vi "Insert Panel to Subpanel.vi"(7 "SubPanel in":refnum<vi>, 8 "error in":errorcluster, 11 "VI Ref":refnum<vi>) -> (0 "error out":errorcluster)   [LabVIEW 2021]
doc: "This vi helps to insert graph or chart vi ref into a subpanel."
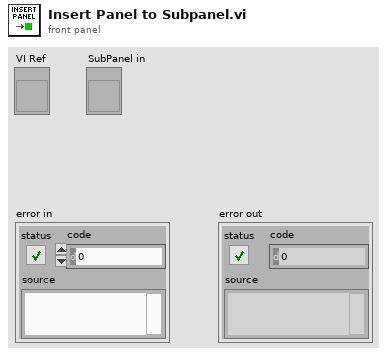
[diagram p1: front panel]
types:
  T1 = enum32{"Invalid", "Standard", "Closed", "Hidden", "Minimized", "Maximized"}
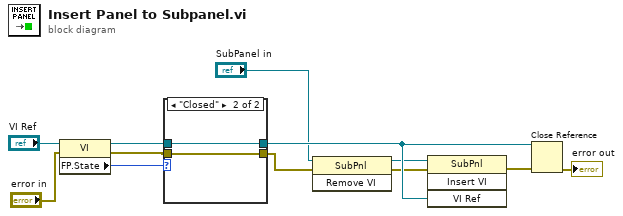
[diagram p0: block diagram]
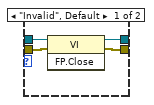
[diagram p2: hidden frame]
diagram:
  n1 = property on="Property Node" class="VI"(reference="VI Ref", error in="error in") -> (reference out=w8:refnum<vi>, error out=w9:errorcluster, "FP.State"=w7:T1)
  n2 = case shown="\"Closed\"" w7 {
    tunnel: [w14 w18] -> w11
    tunnel: [w13 w17] -> w1
    tunnel: w8 -> [w16 w18]
    tunnel: w9 -> [w15 w17]
    frame "Invalid", Default {
      n3 = invoke on="Invoke Node" class="VI" method="FP.Close"(reference=w16, error in=w15) -> (reference out=w14:refnum<vi>, error out=w13:errorcluster)  [unwired: 1 in, 1 out]
    }
    frame "Closed" {
    }
  }
  n4 = invoke on="Invoke Node" class="SubPnl" method="Remove VI"(reference="SubPanel in", error in=w1) -> (reference out=w3:refnum<vi>, error out=w2:errorcluster)  [unwired: 1 in, 1 out]
  n5 = invoke on="Invoke Node" class="SubPnl" method="Insert VI"(reference=w3, error in=w2, "VI Ref"=w11) -> (error out=w10:errorcluster)  [unwired: 1 in, 3 out]
  n6 = Close Reference(reference=w11, error in (no error)=w10) -> (error out=→"error out":errorcluster)
